vi "monochromatorCommandGetSlitWidth.vi"(8 "error in":errorcluster, 10 "port":i32(ring) items=["ONAXISC", "OFFAXISB", "INPORTA"], 11 "monochromator":refnum<k24>) -> (0 "error out":errorcluster, 2 "width":i32, 3 "monochromator":refnum<k24>)   [LabVIEW 2009]
doc: "Get Current Filter"
uses:
  C:/Users/anderson.chen/Desktop/Software Development/Cornerstone Series API (LV9)/Cornerstone DLL/Cornerstone.dll
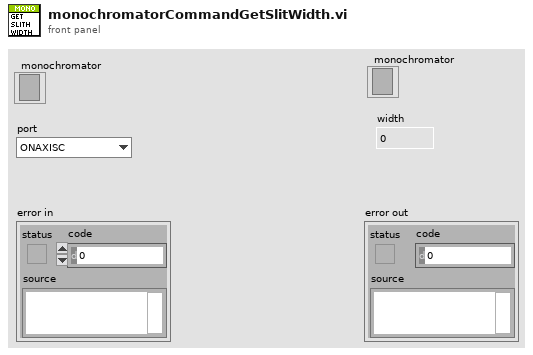
[diagram p1: front panel]
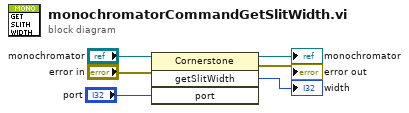
[diagram p0: block diagram]
diagram:
  n1 = invoke class="Cornerstone" method="getSlitWidth"(reference="monochromator", error in="error in", "port"="port") -> (reference out=→"monochromator":refnum<k24>, error out=→"error out":errorcluster, "getSlitWidth"=→"width":i32)  [unwired: 1 in, 1 out]
